vi "SQL_GetRef.vi"(8 "error in (no error)":errorcluster, 11 "reference in":refnum<class "SQL.lvclass">) -> (0 "error out":errorcluster, 3 "reference out":refnum<class "SQL.lvclass">)   [LabVIEW 2012, in "SQL.lvclass"]
uses:
  SQL.lvclass
  <vilib>/addons/database/Connection.llb/Conn ObjectReference.ctl
  <vilib>/addons/database/NI_Database_API.lvlib
panel:
  out "DB Connection Reference":T1
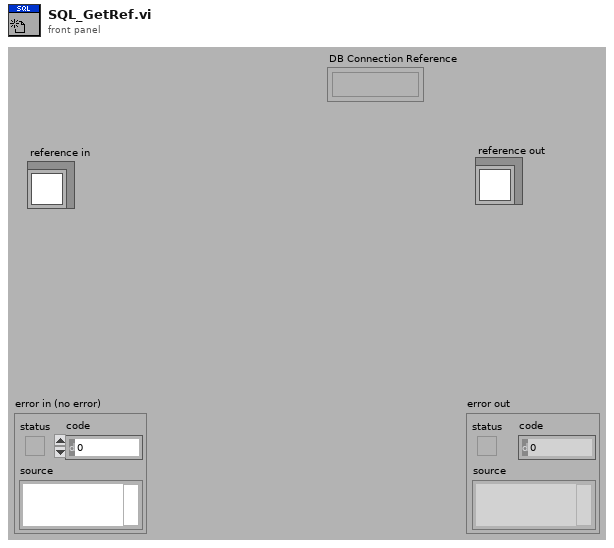
[diagram p1: front panel]
types:
  T1 = typedef "NI_Database_API.lvlib/Conn ObjectReference.ctl" = refnum<k1>
  T2 = typedef "SQL.lvclass/ObjectAttributes.ctl" = cluster{"DB Connection Reference":T1}
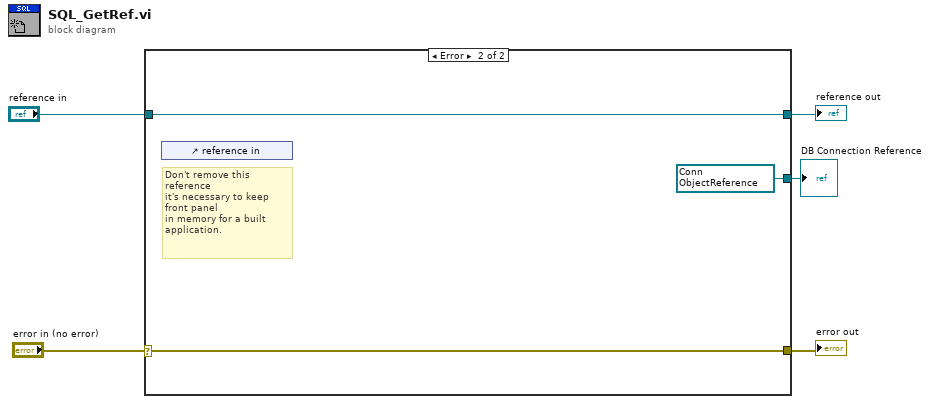
[diagram p0: block diagram]
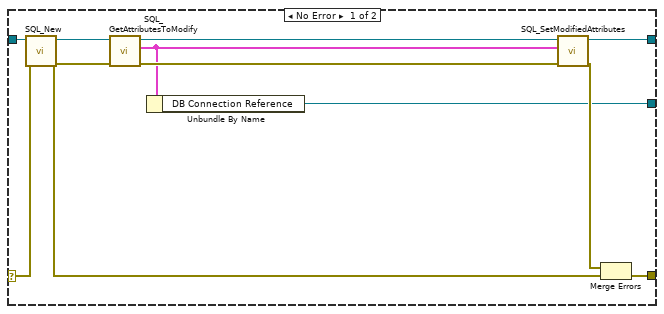
[diagram p2: hidden frame]
diagram:
  n1 = case shown="Error" "error in (no error)" {
    selector: "error in (no error)" -> [w16 w19]
    tunnel: [w10 w19] -> w5
    tunnel: "reference in" -> [w12 w18]
    tunnel: [w13 w18] -> w3
    tunnel: [w6 w17] -> w1
    frame No Error {
      n2 = call "SQL_New.vi"("error in (no error)"=w16, "reference in"=w12) -> ("error out"=w8:errorcluster, "reference out"=w11:refnum<class "SQL.lvclass">)  [unwired: 6 in, 2 out]
      n3 = call "SQL_GetAttributesToModify.vi"("error in (no error)"=w8, "reference in"=w11) -> ("error out"=w15:errorcluster, "Attributes"=w7:T2, "reference out"=w14:refnum<class "SQL.lvclass">)  [unwired: 6 in, 1 out]
      n4 = Unbundle By Name(w7) -> ("DB Connection Reference"=w6:T1)
      n5 = call "SQL_SetModifiedAttributes.vi"("error in (no error)"=w15, "Attributes"=w7, "reference in"=w14) -> ("error out"=w9:errorcluster, "reference out"=w13:refnum<class "SQL.lvclass">)  [unwired: 7 in]
      n6 = Merge Errors(w9, w8) -> (w10:errorcluster)
    }
    frame Error {
      w17 = T1 refnum items=["Connection"] ("DB Connection Reference")
      # "Don't remove this reference\nit's necessary to keep front panel\nin memory for a built application."
      n7 = control-ref of="reference in"() -> ()  [unwired: 1 out]
    }
  }
  "error out" <- w5
  "reference out" <- w3
  "DB Connection Reference" <- w1
